vi "Labview_demo.vi"() -> ()   [LabVIEW 2021]
panel:
  out "Date":string
  out "Nombre de clic":dbl
  in  "Ajouter":bool
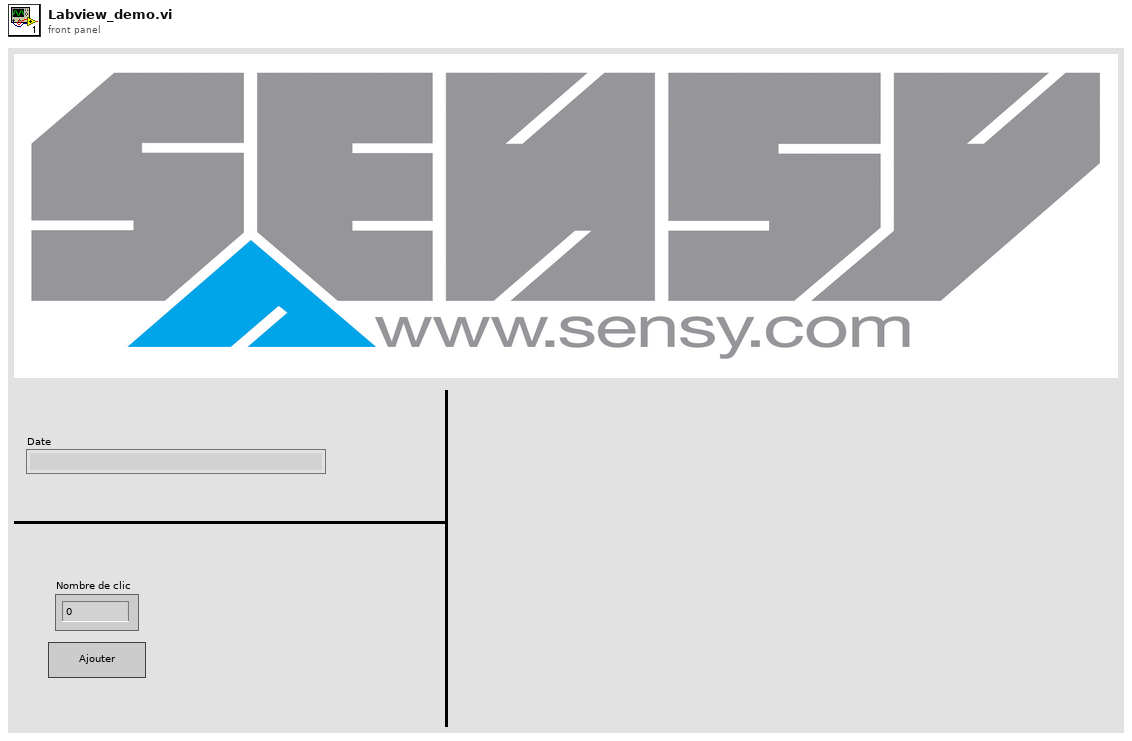
[diagram p1: front panel]
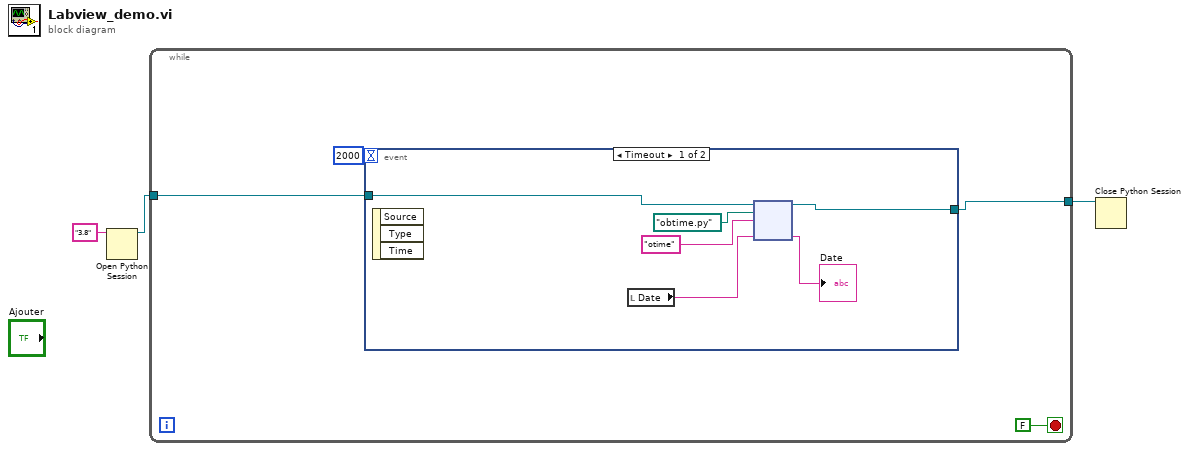
[diagram p0: block diagram]
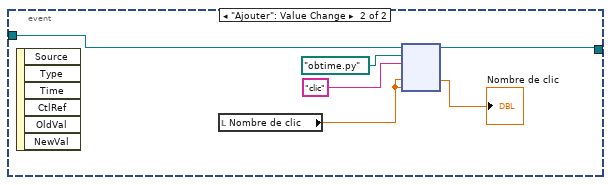
[diagram p2: hidden frame]
diagram:
  n1 = Open Python Session(python version="3.8" ("version Python")) -> (session out=w2:refnum<k35>)  [unwired: 2 in, 1 out]
  n2 = while {
    tunnel: w2 -> [w5]
    tunnel: [w4] -> w1
    stop <- FALSE stop-if-true
    n3 = event shown="[0] Timeout" {
      selector: _ -> [_ _]
      dyn-events: _ -> [_ _]
      timeout: 2000 -> [_ _]
      tunnel: w5 -> [w13 w16]
      tunnel: [w10 w17] -> w4
      event Timeout {
        n4 = event-data() -> ()  [unwired: 1 in, 3 out]
        n5 = local read "Date"() -> (w9:string)
        n6 = node(w13, path "obtime.py" ("chemin du module"), "otime" ("nom de la fonction"), w9) -> (w10:refnum<k35>, →"Date":string)  [unwired: 1 in, 3 out]
      }
      event "Ajouter": Value Change {
        n7 = event-data() -> ()  [unwired: 1 in, 6 out]
        n8 = local read "Nombre de clic"() -> (w14:dbl)
        n9 = node(w16, path "obtime.py" ("chemin du module"), "clic" ("nom de la fonction"), w14, w14) -> (w17:refnum<k35>, →"Nombre de clic":dbl)  [unwired: 2 in, 3 out]
      }
    }
  }
  n10 = Close Python Session(session in=w1) -> ()  [unwired: 1 in, 1 out]
